vi "LU Factorization.vi"   [LabVIEW 2024, in "NI_AALPro.lvlib"]
doc: "<p>Performs the LU factorization of <strong>A</strong> so that <strong>PA</strong> = <strong>LU</strong>. Wire data to the <strong>A</strong> input to determine the polymorphic instance to use or <a href=\"nihelplauncher://docs/csh?context=lvcore_lvhowto_selectingdefaultinstpolyvi\">manually select</a> the instance.</p>"
uses:
  NI_AALPro.lvlib
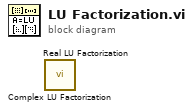
[diagram p0: block diagram]
diagram:
  n1 = call "Complex LU Factorization.vi"() -> ()  [unwired: 1 in, 4 out]
  n2 = call "Real LU Factorization.vi"() -> ()  [unwired: 1 in, 4 out]
